vi "Read State.vi"(8 "error in (no error)":errorcluster, 11 "Expansion in":refnum<class "Recipes.lvclass">) -> (0 "error out":errorcluster, 2 "State":T1, 3 "Expansion out":refnum<class "Recipes.lvclass">)   [LabVIEW 2017, in "Recipes.lvclass"]
uses:
  Recipes.lvclass
  Type Defs/Recipes State.ctl
  Recipes.lvclass/Recipes.ctl
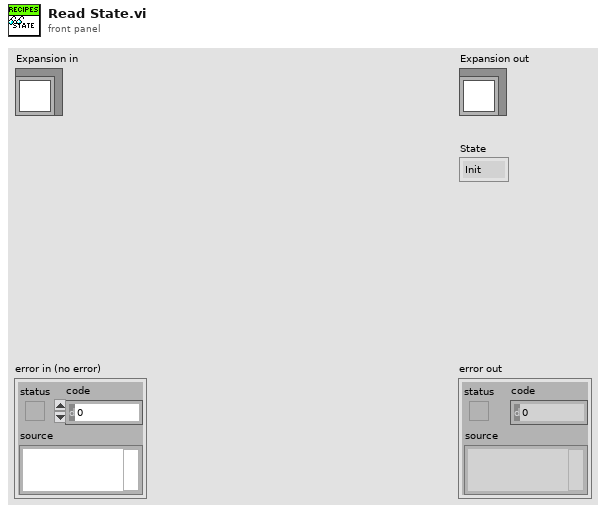
[diagram p1: front panel]
types:
  T1 = typedef "Recipes.lvclass/Recipes State.ctl" = enum16{"Init", "Go", "Stop", "Idle", "Error", "Shutdown"}
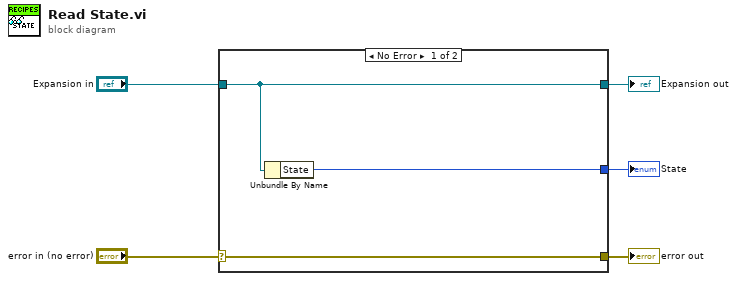
[diagram p0: block diagram]
diagram:
  n1 = case shown="No Error" "error in (no error)" {
    selector: "error in (no error)" -> [w8 w9]
    tunnel: [w8 w9] -> w4
    tunnel: [w7 w10] -> w2
    tunnel: "Expansion in" -> [w7 w10]
    tunnel: [w6 _] -> w1
    frame No Error {
      n2 = Unbundle By Name(w7) -> ("State"=w6:T1)
    }
    frame Error {
    }
  }
  "error out" <- w4
  "Expansion out" <- w2
  "State" <- w1
